vi "Init Shared Variable.vi"(8 "error in":errorcluster, 11 "name":string) -> (0 "error out 2":errorcluster)   [LabVIEW 2017, in "Status Monitor Library.lvlib"]
uses:
  Status Monitor Library.lvlib
  Network Shared Variables/Shared Variables Library.lvlib
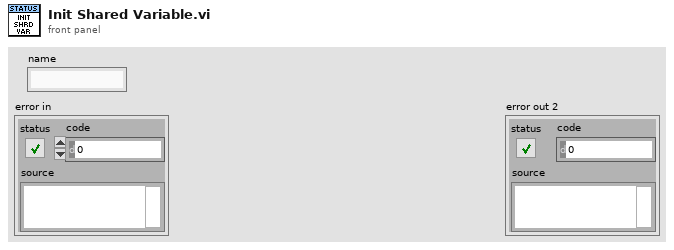
[diagram p1: front panel]
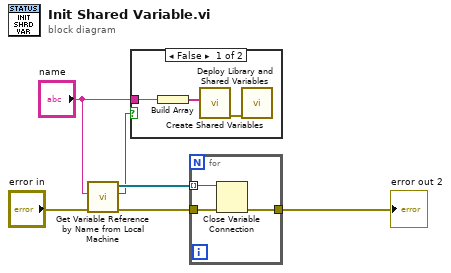
[diagram p0: block diagram]
diagram:
  n1 = call "Get Variable Reference by Name from Local Machine.vi"("error in"="error in", "Search"="name") -> ("error out"=w4:errorcluster, "Found"=w5:bool, "Variable References Out"=w6:refnum<k21>[])  [unwired: 7 in]
  n2 = case shown="False" w5 {
    tunnel: "name" -> [w7 _]
    frame False {
      n3 = Build Array(w7) -> (w8:string[])
      n4 = call "Create Shared Variables.vi"("Variable Names"=w8) -> ("error out"=w9:errorcluster)  [unwired: 10 in]
      n5 = call "Deploy Library and Shared Variables.vi"("error in"=w9) -> ()  [unwired: 10 in, 1 out]
    }
    frame True {
    }
  }
  n6 = for {
    tunnel: w6 -> [w12] mode=indexing
    tunnel: w4 -> [w11]
    tunnel: [w10] -> w1
    n7 = Close Variable Connection(8:w11, 11:w12) -> (0:w10:errorcluster)
  }
  "error out 2" <- w1
